vi "get enum reference.vi"(8 "error in":errorcluster, 11 "test displayable in":refnum<class "test displayable.lvclass">) -> (0 "error out":errorcluster, 2 "enum":variant, 3 "test displayable out":refnum<class "test displayable.lvclass">)   [LabVIEW 2013, in "test displayable.lvclass"]
uses:
  test displayable.lvclass
  properties.ctl
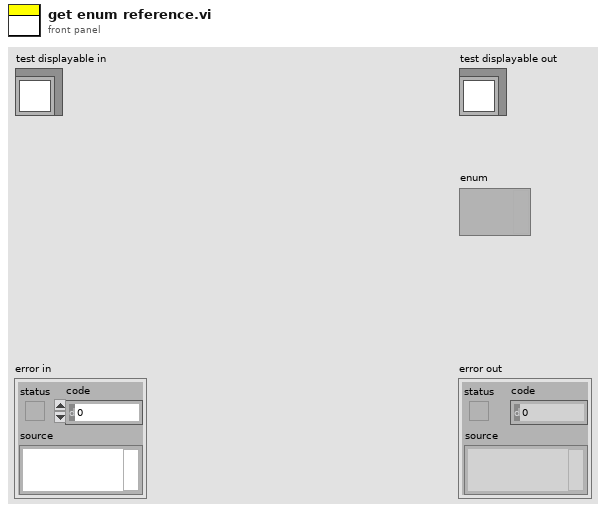
[diagram p1: front panel]
types:
  T1 = typedef "test displayable.lvclass/properties.ctl" = enum16{"1", "2"}
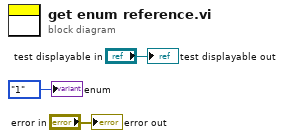
[diagram p0: block diagram]
diagram:
  "error out" <- "error in"
  "test displayable out" <- "test displayable in"
  "enum" <- properties."1" ("props")
